vi "Add Capabilities.vi"(8 "error in (no error)":errorcluster, 10 "Capabilities":string[](array[string]), 11 "Node Config in":refnum<class "Node Config.lvclass">) -> (0 "error out":errorcluster, 3 "Node Config out":refnum<class "Node Config.lvclass">)   [LabVIEW 2020, in "Vecto.lvlib" / "Node Config.lvclass"]
uses:
  Node Config.lvclass
  Node Config.lvclass/Node Config.ctl
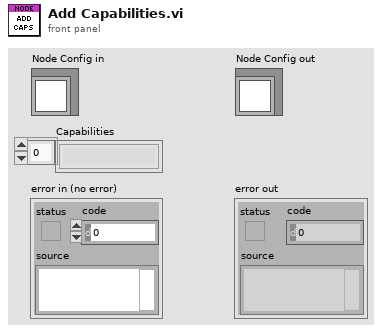
[diagram p1: front panel]
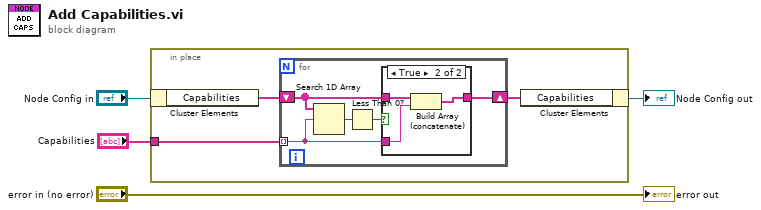
[diagram p0: block diagram]
diagram:
  n1 = in-place {
    in-place-border: "Capabilities" -> [w6]
    n2 = in-place-cluster #1("Node Config in") -> ("Capabilities"=w7:string[])
    n3 = for {
      shift-right: [w9] -> w5
      shift-left: w7 -> [w11]
      tunnel: w6 -> [w8] mode=indexing
      n4 = Search 1D Array(1D array=w11, element=w8) -> (index of element=w12:i32)  [unwired: 1 in]
      n5 = Less Than 0?(x=w12) -> (x < 0?=w10:bool)
      n6 = case shown="True" w10 {
        tunnel: w11 -> [w13 w16]
        tunnel: [w13 w14] -> w9
        tunnel: w8 -> [_ w15]
        frame False {
        }
        frame True {
          n7 = Build Array (concatenate)(w16, w15) -> (w14:string[])
        }
      }
    }
    n8 = in-place-cluster #1("Capabilities"=w5) -> (→"Node Config out":refnum<class "Node Config.lvclass">)
  }
  "error out" <- "error in (no error)"
